vi "Write to TDMS File.vi"(6 "Waveforms":waveform(sgl)[](array[waveform]), 7 "Time Stamp":timestamp, 8 "error in (no error)":errorcluster, 9 "Frequency":dbl[](array[numeric]), 10 "Amplitude":dbl[](array[numeric]), 11 "Damping":dbl[](array[numeric])) -> (0 "error out":errorcluster)   [LabVIEW 2013]
doc: "Statnett PMU Reference Library\nWirtes data to TDMS File"
panel:
  in  "TDMS File Path":path=path "\\\\oslfp1.statnett.no\\Users/jukkat/testfile.tdms"
  # "INPUT"
  # "INTERMEDIATE"
  # "OUTPUT"
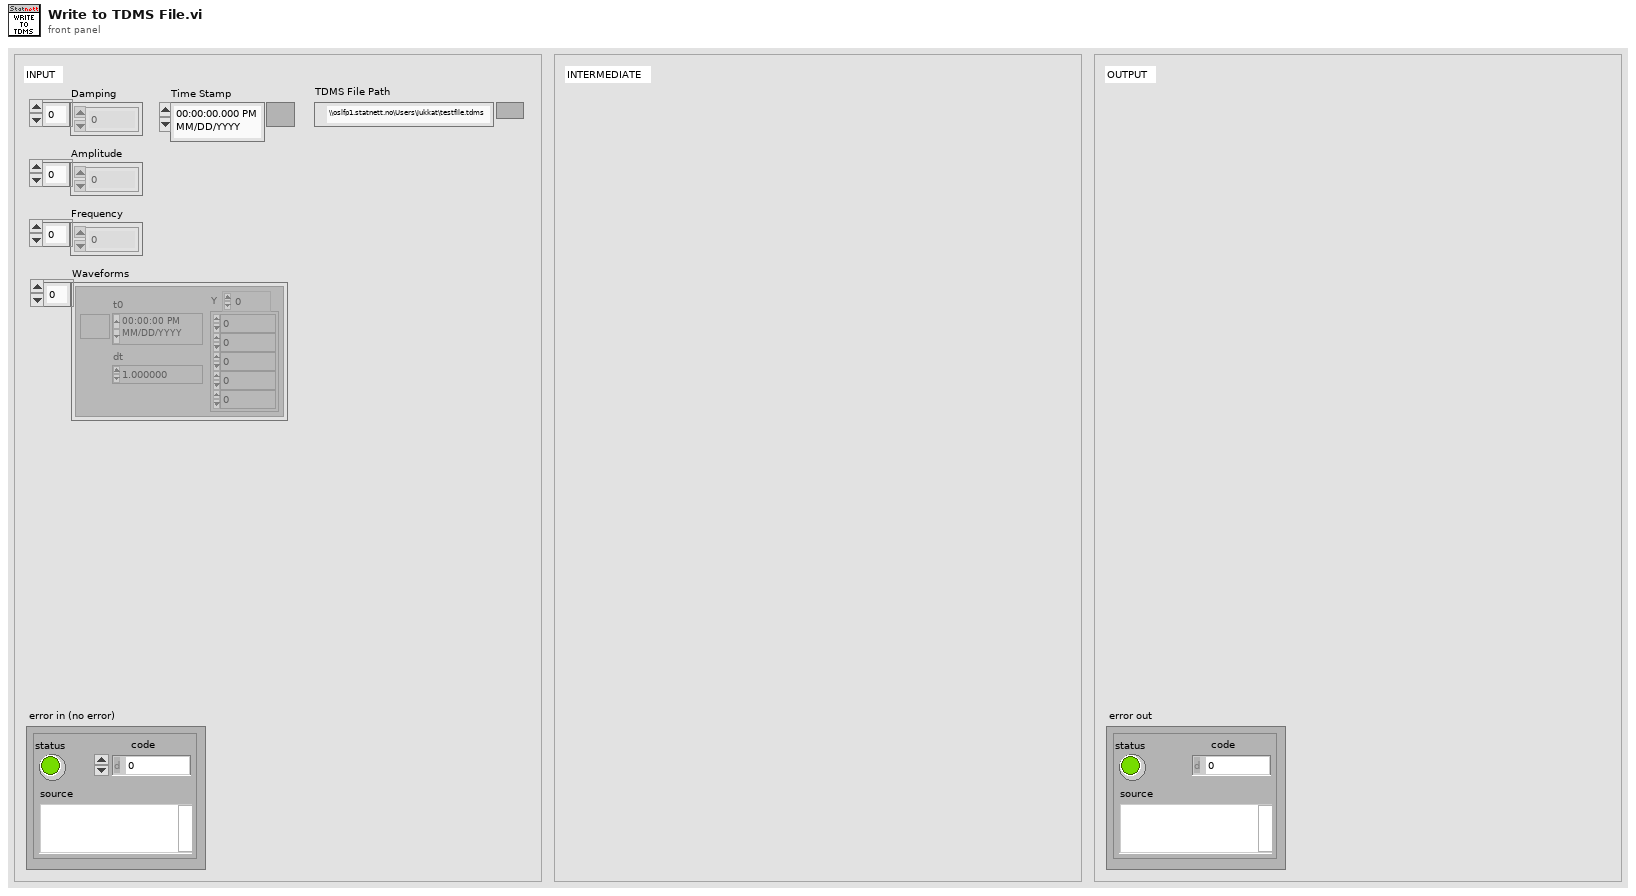
[diagram p1: front panel]
types:
  T1 = enum16{"open", "open or create", "create or replace", "create", "open (read-only)"}
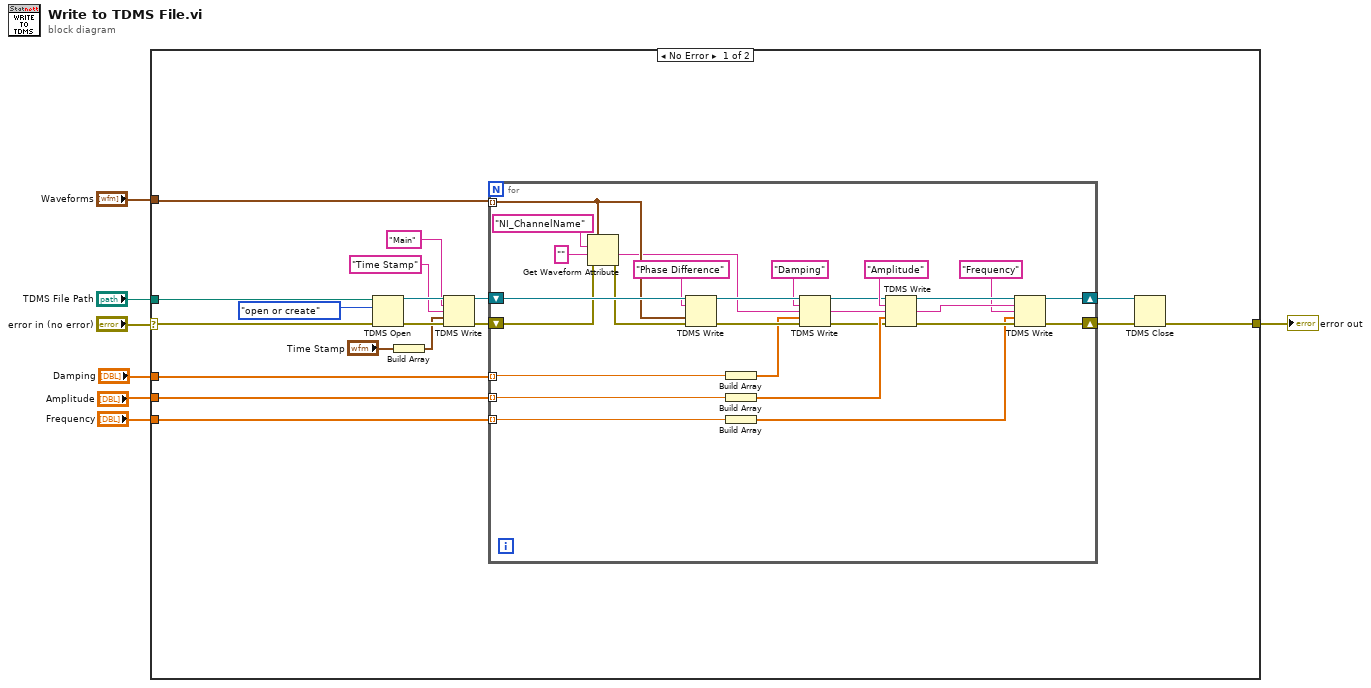
[diagram p0: block diagram]
diagram:
  n1 = case shown="No Error" "error in (no error)" {
    selector: "error in (no error)" -> [w9 w51]
    tunnel: [w8 w51] -> w6
    tunnel: "Waveforms" -> [w14 _]
    tunnel: "TDMS File Path" -> [w13 _]
    tunnel: "Damping" -> [w12 _]
    tunnel: "Amplitude" -> [w11 _]
    tunnel: "Frequency" -> [w10 _]
    frame No Error {
      n2 = TDMS Open(8:w9, 10:T1."open or create" ("operation (0:open)"), 11:w13) -> (0:w21:errorcluster, 3:w22:refnum<k34>)  [unwired: 4 in]
      n3 = Build Array("Time Stamp") -> (w17:timestamp[])
      n4 = TDMS Write(0:w22, 5:"Main" ("group name in (Untitled)"), 7:"Time Stamp" ("group name in (Untitled)"), 9:w17, 11:w21) -> (4:w24:refnum<k34>, 15:w23:errorcluster)  [unwired: 1 in, 2 out]
      n5 = for {
        tunnel: w14 -> [w46] mode=indexing
        tunnel: w12 -> [w42] mode=indexing
        tunnel: w11 -> [w38] mode=indexing
        tunnel: w10 -> [w31] mode=indexing
        shift-right: [w29] -> w16
        shift-left: w24 -> [w50]
        shift-right: [w28] -> w15
        shift-left: w23 -> [w27]
        n6 = Get Waveform Attribute(4:w27, 5:"" ("name"), 6:"NI_ChannelName" ("name"), 7:w46) -> (0:w26:errorcluster, 1:w33:string)  [unwired: 2 out]
        n7 = TDMS Write(0:w50, 5:"Phase Difference" ("group name in (Untitled)"), 9:w46, 11:w26) -> (4:w48:refnum<k34>, 15:w47:errorcluster)  [unwired: 2 in, 2 out]
        n8 = Build Array(w42) -> (w41:dbl[])
        n9 = Build Array(w38) -> (w37:dbl[])
        n10 = Build Array(w31) -> (w30:dbl[])
        n11 = TDMS Write(0:w48, 5:"Damping" ("group name in (Untitled)"), 7:w33, 9:w41, 11:w47) -> (4:w39:refnum<k34>, 15:w36:errorcluster)  [unwired: 1 in, 2 out]
        n12 = TDMS Write(0:w39, 5:"Amplitude" ("group name in (Untitled)"), 7:w33, 9:w37, 11:w36) -> (4:w35:refnum<k34>, 15:w34:errorcluster)  [unwired: 1 in, 2 out]
        n13 = TDMS Write(0:w35, 5:w33, 7:"Frequency" ("group name in (Untitled)"), 9:w30, 11:w34) -> (4:w29:refnum<k34>, 15:w28:errorcluster)  [unwired: 1 in, 2 out]
      }
      n14 = TDMS Close(8:w15, 11:w16) -> (0:w8:errorcluster)  [unwired: 1 out]
    }
    frame Error {
    }
  }
  "error out" <- w6
